vi "SwitchTest.vi"() -> ()   [LabVIEW 2009]
uses:
  Packet.ctl
panel:
  out "Switches":u8 format="%.0b"
  out "HexKeys":u8=212 format="%.0x"
  in  "stop":bool
  in  "VISA resource name":refnum<visa-resource-name>="COM15"
  out "error out":errorcluster
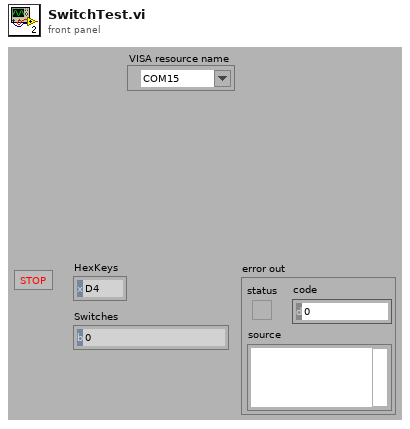
[diagram p1: front panel]
types:
  T1 = typedef "Packet.ctl" = cluster{"Length":u8, "Type":u8, "PID":u8, "Data":u8[], "CRC":u8}
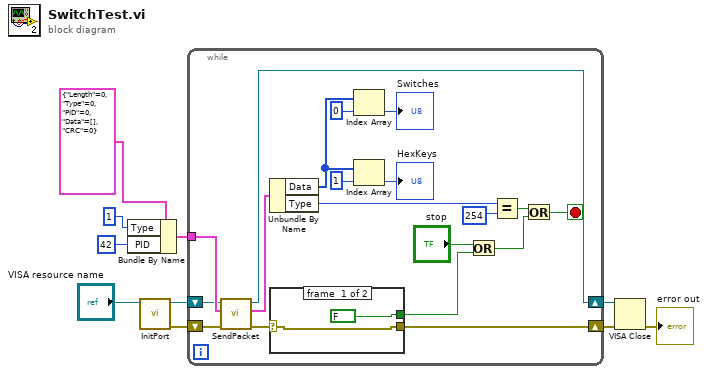
[diagram p0: block diagram]
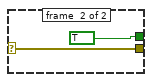
[diagram p2: hidden frame]
diagram:
  n1 = Bundle By Name(cluster=T1 {"Length"=0, "Type"=0, "PID"=0, "Data"=[], "CRC"=0} ("Transmit"), "Type"=u8 1, "PID"=u8 42) -> (w5:T1)
  n2 = call "InitPort.vi"("VISA resource name"="VISA resource name") -> ("error out"=w2:errorcluster, "VISA resource name out"=w4:refnum<visa-resource-name>)  [unwired: 9 in]
  n3 = while {
    tunnel: w5 -> [w29]
    shift-right: [w27] -> w3
    shift-left: w4 -> [w28]
    shift-right: [w23] -> w1
    shift-left: w2 -> [w26]
    stop <- w17 stop-if-true
    n4 = call "SendPacket.vi"("error in (no error)"=w26, "Transmit"=w29, "VISA resource name"=w28) -> ("error out"=w24:errorcluster, "Response"=w25:T1, "VISA resource name out"=w27:refnum<visa-resource-name>)  [unwired: 6 in]
    n5 = Unbundle By Name(w25) -> ("Data"=w15:u8[], "Type"=w20:u8)
    n6 = case shown="No Error" w24 {
      selector: w24 -> [w30 w33]
      tunnel: [w30 w33] -> w23
      tunnel: [FALSE TRUE] -> w22
      frame #0 {
      }
      frame #1 {
      }
    }
    n7 = Index Array(array=w15, index=0) -> (element=→"Switches":u8)
    n8 = Index Array(array=w15, index=1) -> (element=→"HexKeys":u8)
    n9 = Or(x="stop", y=w22) -> (x .or. y?=w18:bool)
    n10 = Equal?(x=w20, y=u8 254) -> (x = y?=w16:bool)
    n11 = Or(x=w16, y=w18) -> (x .or. y?=w17:bool)
  }
  n12 = VISA Close(VISA resource name=w3, error in (no error)=w1) -> (error out=→"error out":errorcluster)
